vi "SpoldrxPwr.vi"(6 "SpecifyTypeOfDataAcq":string="_", 8 "error in (no error)":errorcluster, 9 "startGate":i32=200 min=1025 step=1, 10 "nGates":i32=500 min=1025 step=1, 11 "nSamples":i32=1000) -> (0 "Comm error":errorcluster, 1 "XML error":errorcluster, 2 "String_of_drx_Powers":string, 3 "drx_power":T1 {"time" format="%<%H:%M:%S\n%Y/%m/%d>T"})   [LabVIEW 2012]
doc: "Reads the power from the N1911A power meter."
uses:
  drxPowerData.ctl
panel:
  out "XML Response":string="fetch?"
  out "XML commands":string="<TsGrabberCommands>\n  <nSamples>1000</nSamples>\n  <startGate>50</startGate>\n  <nGates>500</nGates>\n  <fastAlternating>true</fastAlternating>\n  <labviewRequest>true</labviewRequest>\n</TsGrabberCommands>\n"
  # "Changed StartGate and nGates to I32 and corrected wiring to each of these (fp:17Aug07).  The defaults must be 1000/500/50 for the calibration programs to work correctly!"
  # "Select ngates and startgate to avoid standard test pulse and Rx switching transient"
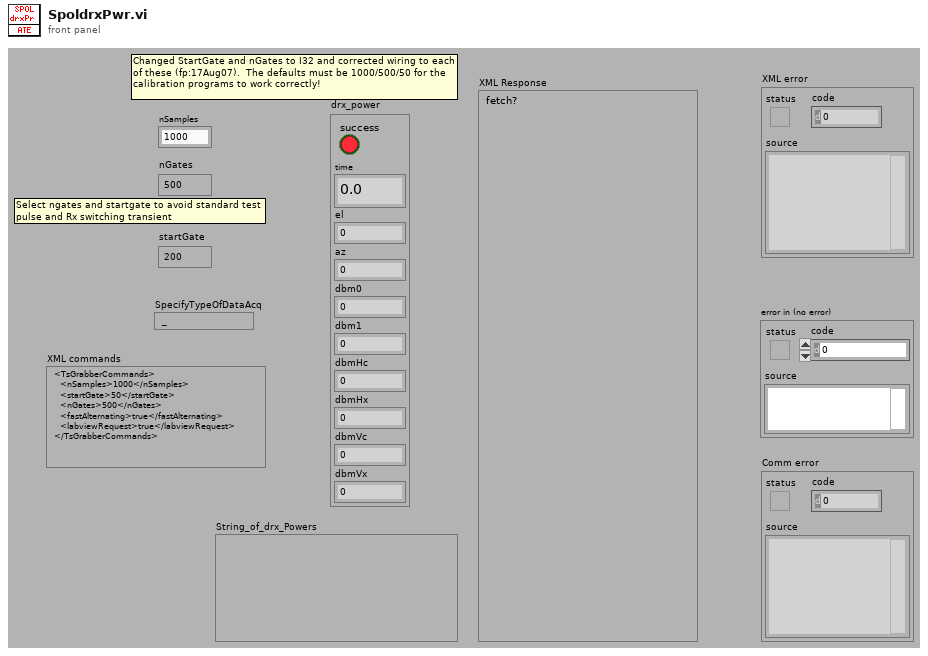
[diagram p1: front panel]
types:
  T1 = typedef "drxPowerData.ctl" = cluster{"success":bool, "time":dbl, "el":dbl, "az":dbl, "dbm0":dbl, "dbm1":dbl, "dbmHc":dbl, "dbmHx":dbl, "dbmVc":dbl, "dbmVx":dbl}
  T2 = enum16{"N1911A", "Siggen", "34980a", "E4418B", "Rvp8", "spoldrx"}
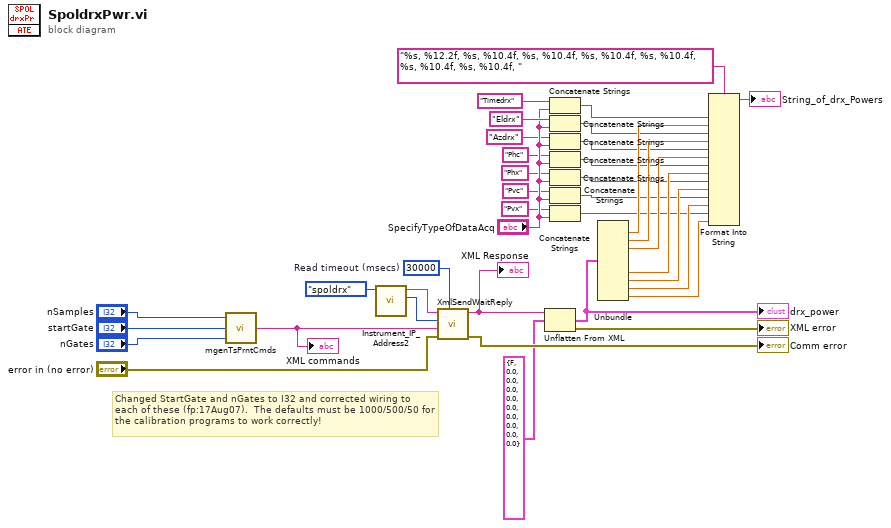
[diagram p0: block diagram]
diagram:
  w35 = 30000  # Read timeout (msecs)
  # "Changed StartGate and nGates to I32 and corrected wiring to each of these (fp:17Aug07).  The defaults must be 1000/500/50 for the calibration programs to work correctly!"
  n1 = call "mgenTsPrntCmds.vi"("nGates"="nGates", "startGate"="startGate", "nSamples"="nSamples") -> ("TsPrintCommand"=w5:string)
  "XML commands" <- w5
  n2 = call "Instrument_IP_Address2.vi"("Instrument"=T2."spoldrx") -> ("Port"=w37:u16, "IP Address"=w36:string)  [unwired: 9 in]
  n3 = call "XmlSendWaitReply.vi"("Read timeout msecs"=w35, "error in (no error)"="error in (no error)", "Command"=w5, "TCP port"=w37, "IP Address"=w36) -> ("Error out"=→"Comm error":errorcluster, "Reply"=w7:string)  [unwired: 4 in]
  "XML Response" <- w7
  n4 = Unflatten From XML(xml string=w7, type=T1 {"success"=FALSE, "time"=0.0, "el"=0.0, "az"=0.0, "dbm0"=0.0, "dbm1"=0.0, "dbmHc"=0.0, "dbmHx"=0.0, "dbmVc"=0.0, "dbmVx"=0.0} ("drx cluster")) -> (value=w31:T1, error out=→"XML error":errorcluster)  [unwired: 1 in]
  "drx_power" <- w31
  n5 = Concatenate Strings("Timedrx", "SpecifyTypeOfDataAcq") -> (w17:string)
  n6 = Concatenate Strings("Eldrx", "SpecifyTypeOfDataAcq") -> (w16:string)
  n7 = Concatenate Strings("Azdrx", "SpecifyTypeOfDataAcq") -> (w15:string)
  n8 = Concatenate Strings("Phc", "SpecifyTypeOfDataAcq") -> (w13:string)
  n9 = Concatenate Strings("Phx", "SpecifyTypeOfDataAcq") -> (w12:string)
  n10 = Concatenate Strings("Pvc", "SpecifyTypeOfDataAcq") -> (w11:string)
  n11 = Concatenate Strings("Pvx", "SpecifyTypeOfDataAcq") -> (w10:string)
  n12 = Unbundle(w31) -> ("time"=w30:dbl, "el"=w29:dbl, "az"=w14:dbl, "dbmHc"=w28:dbl, "dbmHx"=w27:dbl, "dbmVc"=w26:dbl, "dbmVx"=w25:dbl)  [unwired: 3 out]
  n13 = Format Into String(format string="%s, %12.2f, %s, %10.4f, %s, %10.4f, %s, %10.4f, %s, %10.4f, %s, %10.4f, %s, %10.4f, ", w17, w30, w16, w29, w15, w14, w13, w28, w12, w27, w11, w26, w10, w25) -> (resulting string=→"String_of_drx_Powers":string)  [unwired: 2 in, 1 out]
